vi "Read Map.vi"(8 "error in (no error)":errorcluster, 11 "JobReport in":refnum<class "JobReport.lvclass">) -> (0 "error out":errorcluster, 2 "Map":variant, 3 "JobReport out":refnum<class "JobReport.lvclass">)   [LabVIEW 2013, in "openCronJob.lvlib" / "JobReport.lvclass"]
uses:
  JobReport.lvclass
  JobReport.lvclass/JobReport.ctl
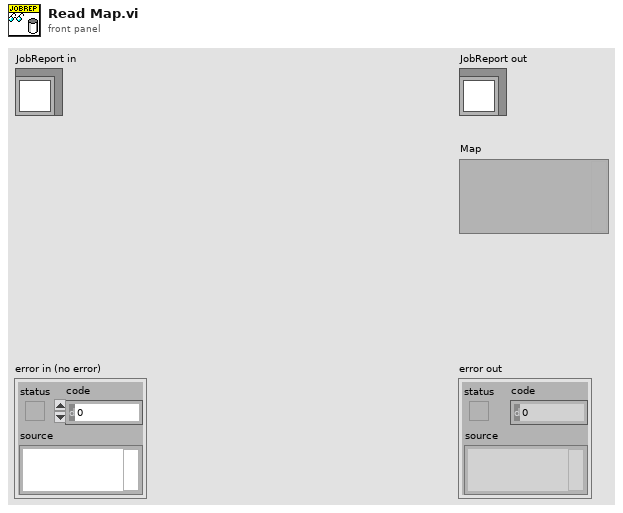
[diagram p1: front panel]
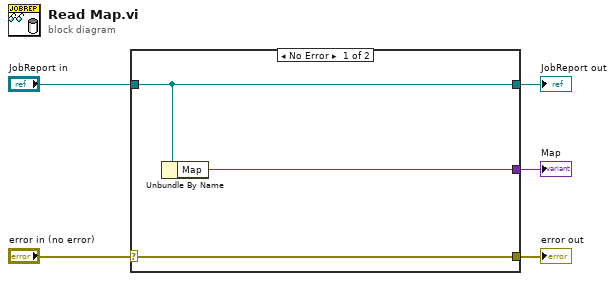
[diagram p0: block diagram]
diagram:
  n1 = case shown="No Error" "error in (no error)" {
    selector: "error in (no error)" -> [w8 w9]
    tunnel: [w8 w9] -> w4
    tunnel: [w7 w10] -> w2
    tunnel: "JobReport in" -> [w7 w10]
    tunnel: [w6 _] -> w1
    frame No Error {
      n2 = Unbundle By Name(w7) -> ("Map"=w6:variant)
    }
    frame Error {
    }
  }
  "error out" <- w4
  "JobReport out" <- w2
  "Map" <- w1
